vi "DISP_WIND_ANN_MARK_STAT.vi"(0 "VISA IN":refnum<visa-resource-name>, 1 "ON | OFF":bool, 5 "error in":errorcluster, 7 "Window":i32) -> (14 "VISA Out":refnum<visa-resource-name>, 19 "error out":errorcluster)   [LabVIEW 2018, in "PNA-X.lvlib"]
doc: "DISPlay:WINDow<wnum>:ANNotation:MARKer:STATe <ON | OFF> \n(Read-Write) Specifies whether to show or hide the Marker readout (when markers are ON) on the \nselected window. See other SCPI Marker commands. Learn more about Marker readout. \nParameters \n<wnum> Any existing window number. If unspecified, value is set to 1. \n<ON | OFF> ON (or 1) - turns marker readout ON. \nOFF (or 0) - turns marker readout OFF. \nExamples DISP:WIND:ANN:MARK:STAT ON \ndisplay:window:annotation:marker:state off \nQuery Syntax DISPlay:WINDow:ANNotation:MARKer:STATe? \nReturn Type Boolean (1 = ON, 0 = OFF) \nDefault ON"
uses:
  PNA-X.lvlib
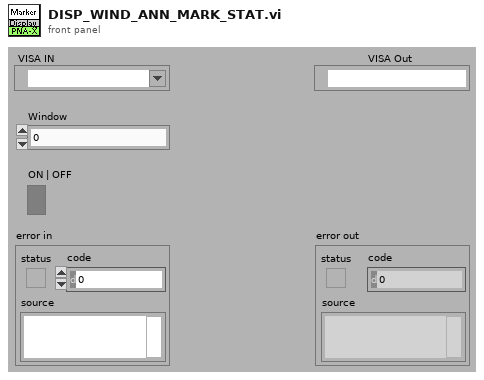
[diagram p1: front panel]
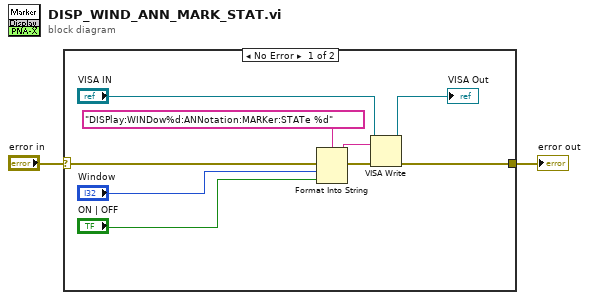
[diagram p0: block diagram]
diagram:
  n1 = case shown="No Error" "error in" {
    selector: "error in" -> [w11 w12]
    tunnel: [w6 w12] -> w1
    frame No Error {
      n2 = Format Into String(format string="DISPlay:WINDow%d:ANNotation:MARKer:STATe %d" ("Cmdline"), error in=w11, "Window", "ON | OFF") -> (resulting string=w9:string, error out=w10:errorcluster)  [unwired: 1 in]
      n3 = VISA Write(VISA resource name="VISA IN", write buffer=w9, error in (no error)=w10) -> (VISA resource name out=→"VISA Out":refnum<visa-resource-name>, error out=w6:errorcluster)  [unwired: 1 out]
    }
    frame Error {
    }
  }
  "error out" <- w1
